vi "test.vi"() -> ()   [LabVIEW 2020]
uses:
  exportDll.dll
panel:
  out "arg2":dbl[](array[numeric])
  in  "n":i32
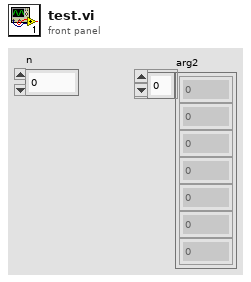
[diagram p1: front panel]
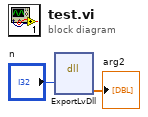
[diagram p0: block diagram]
diagram:
  n1 = dll-call lib="E:/Practice/Lv/dll/CppDllForLv/src/LV/builds/PassingTest/MyDLL/exportDll.dll" fn="ExportLvDll"("n"="n") -> ("arg2"=→"arg2":dbl[])  [unwired: 6 in, 2 out]
